vi "Example Binary.vi"() -> ()   [LabVIEW 2020]
uses:
  <vilib>/Utility/sysdir.llb/System Directory Type.ctl
  Sources/_Helpers/Tiff Page Details.ctl
  Sources/TIFF Writer/TIFF Writer.lvclass
  Sources/LV Tiff.lvlib
panel:
  out "Intensity Graph":u8[][](graph)
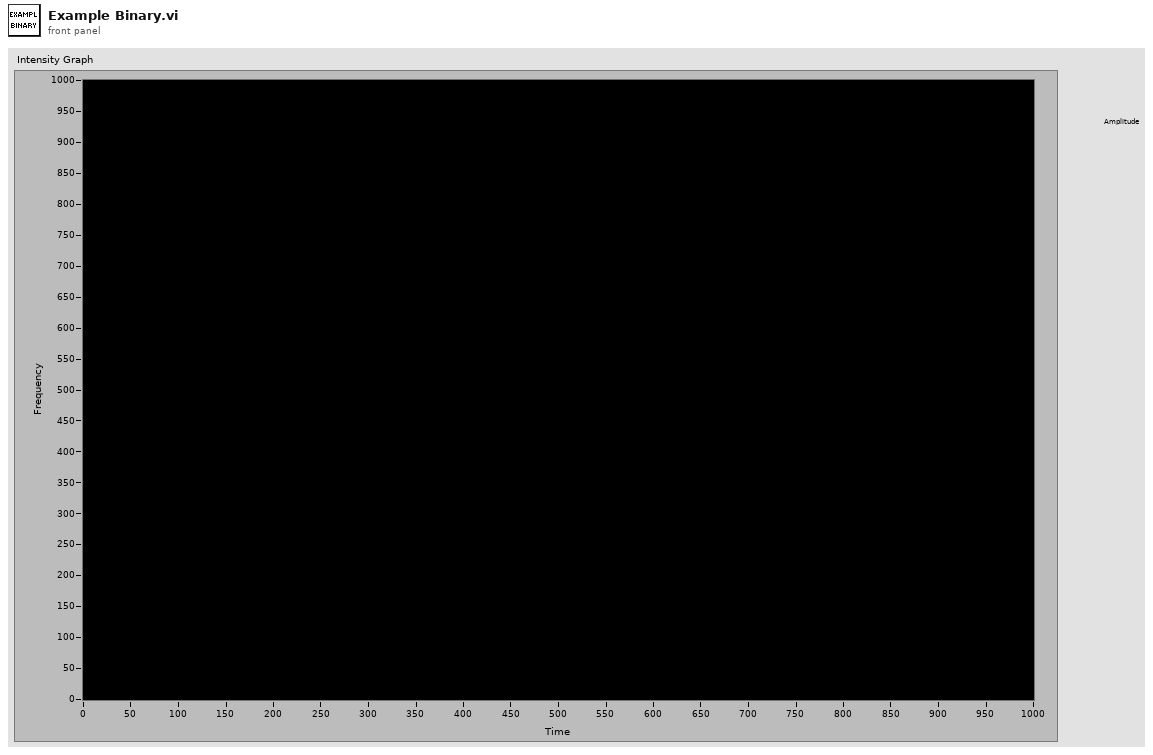
[diagram p1: front panel]
types:
  T1 = typedef "LV Tiff.lvlib/Tiff Page Details.ctl" = cluster{"ImageDescription":string, "XResolution":dbl, "YResolution":dbl, "ResolutionUnit":enum16{"None", "Inch", "Centimeter"}, "PhotometricInterpretation":u16, "Compression":enum16{"None", "Deflate", "JPEG"}, "PageName":string, "DocumentName":string}
  T2 = enum16{"open", "replace", "create", "open or create", "replace or create", "replace or create with confirmation"}
  T3 = typedef "System Directory Type.ctl" = i32
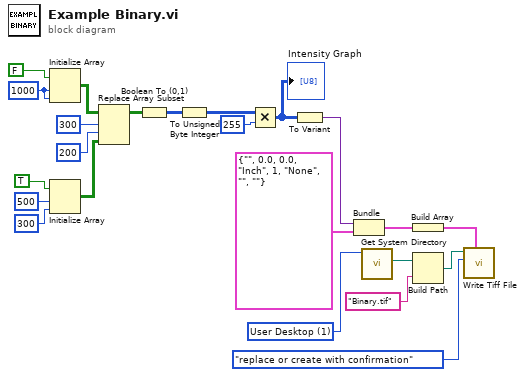
[diagram p0: block diagram]
diagram:
  w23 = T3 1 items=["User Home"=0, "User Desktop"=1, "User Documents"=2, "User Application Data"=3, "User Preferences"=4, "User Temporary"=5, "Public Documents"=6, "Public Application Data"=7, "Public Preferences"=8, "Public Cache"=13, "System Core Libraries"=9, "System Installed Libraries"=10, "Application Files"=11, "Boot Volume Root"=12] ("system directory type")
  w9 = 1000
  n1 = Initialize Array(FALSE, w9, w9) -> (w11:bool[][])
  n2 = Initialize Array(TRUE ("element"), 500 ("dimension size"), 300 ("dimension size")) -> (w3:bool[][])
  n3 = Replace Array Subset(array=w11, new element=w3, index (row)=300, index (col)=200 ("disabled index (col)")) -> (w8:bool[][])
  n4 = Boolean To (0,1)(Boolean=w8) -> (0, 1=w14:i16[][])
  n5 = To Unsigned Byte Integer(number=w14) -> (unsigned 8bit integer=w13:u8[][])
  n6 = Multiply(x=w13, y=u8 255) -> (x*y=w10:u8[][])
  "Intensity Graph" <- w10
  n7 = To Variant(anything=w10) -> (Variant=w18:variant)
  n8 = Bundle("Variant"=w18, "Details"=T1 {"ImageDescription"="", "XResolution"=0.0, "YResolution"=0.0, "ResolutionUnit"=enum."Inch", "PhotometricInterpretation"=1, "Compression"=enum."None", "PageName"="", "DocumentName"=""}) -> (w16:cluster{"Variant":variant, "Details":T1})  [unwired: 1 in]
  n9 = call <vilib>:"Get System Directory.vi"("system directory type"=w23) -> ("system directory"=w22:path)  [unwired: 10 in]
  n10 = Build Array(w16) -> (w15:cluster{"Variant":variant, "Details":T1}[])
  n11 = Build Path(base path=w22, name or relative path="Binary.tif") -> (appended path=w20:path)
  n12 = call "Write Tiff File.vi"("Pages"=w15, "operation (replace)"=T2."replace or create with confirmation", "Path"=w20) -> ()  [unwired: 7 in, 2 out]
